vi "GlobalVISA7.vi"() -> ()   [LabVIEW 2013]
panel:
  in  "VISA resource name":refnum<visa-resource-name>
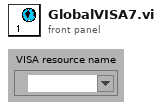
[diagram p1: front panel]
diagram:
